vi "模拟量采集.vi"(11 "STOP 2":bool) -> (0 "压力2":dbl[](array[numeric]) format="%.2f", 1 "位移2":dbl[](array[numeric]) format="%.2f", 2 "压力1":dbl[](array[numeric]) format="%.2f", 3 "位移1":dbl[](array[numeric]) format="%.2f")   [LabVIEW 2010]
panel:
  out "CH0 15":dbl[](array[numeric]) format="%.2f"
  out "CH0 14":dbl[](array[numeric]) format="%.2f"
  out "CH0 13":dbl[](array[numeric]) format="%.2f"
  out "CH0 12":dbl[](array[numeric]) format="%.2f"
  out "CH0 11":dbl[](array[numeric]) format="%.2f"
  out "CH0 10":dbl[](array[numeric]) format="%.2f"
  out "CH0 9":dbl[](array[numeric]) format="%.2f"
  out "CH0 8":dbl[](array[numeric]) format="%.2f"
  out "CH0 7":dbl[](array[numeric]) format="%.2f"
  out "CH0 6":dbl[](array[numeric]) format="%.2f"
  out "CH0 5":dbl[](array[numeric]) format="%.2f"
  out "CH0 4":dbl[](array[numeric]) format="%.2f"
  # "±10V量程采集演示"
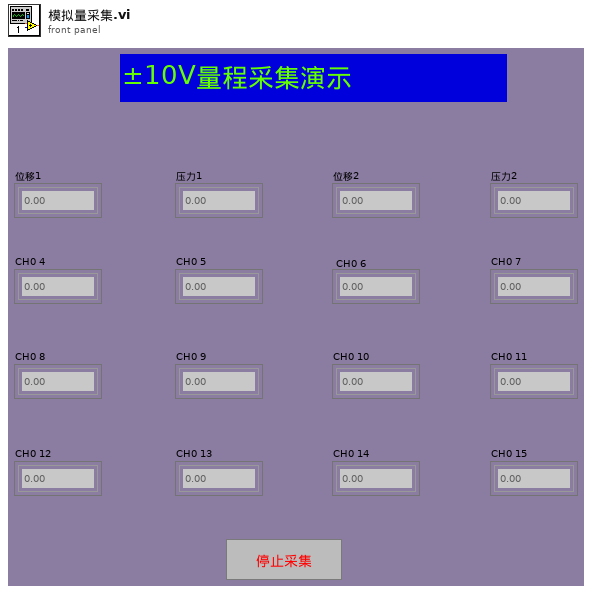
[diagram p1: front panel]
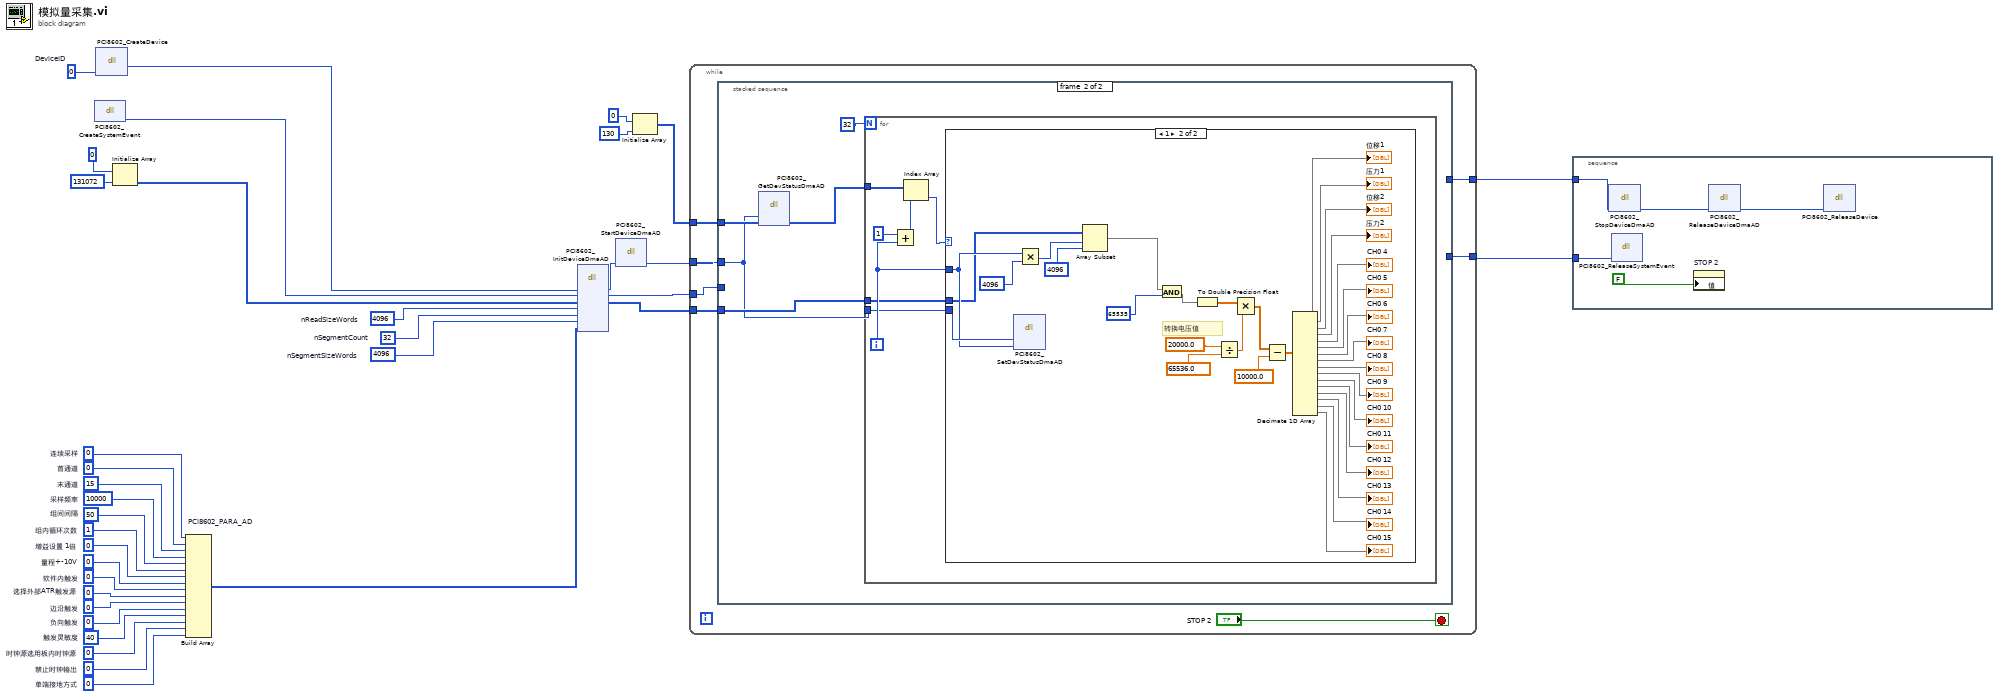
[diagram p0: block diagram]
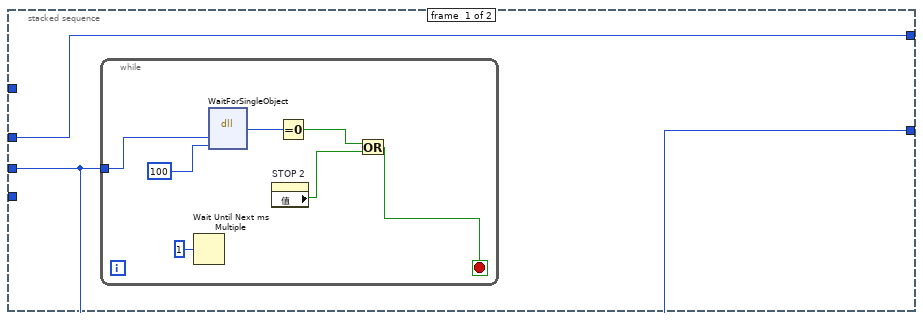
[diagram p2: hidden frame]
diagram:
  w1 = 0  # 单端接地方式
  w4 = 40  # 触发灵敏度
  w10 = 0  # 增益设置 1倍
  w11 = 1  # 组内循环次数
  w12 = 50  # 组间间隔
  w14 = 15  # 末通道
  w15 = 0  # 首通道
  w16 = 0  # 连续采样
  w2 = 0  # 禁止时钟输出
  w3 = 0  # 时钟源选用板内时钟源
  w5 = 0  # 负向触发
  w6 = 0  # 边沿触发
  w7 = 0  # 选择外部ATR触发源
  w8 = 0  # 软件内触发
  w9 = 0  # 量程+-10V
  w13 = 10000  # 采样频率
  w18 = 4096  # nSegmentSizeWords
  w19 = 32  # nSegmentCount
  w20 = 4096  # nReadSizeWords
  w28 = 0  # DeviceID
  n1 = dll-call lib="PCI8602" fn="PCI8602_CreateSystemEvent" label="CreateSystemEvent"() -> ("hEvent"=w22:i32)  [unwired: 3 in, 2 out]
  n2 = dll-call lib="PCI8602" fn="PCI8602_CreateDevice" label="CreateDevice"("DeviceID"=w28) -> (w23:i32)  [unwired: 4 in, 2 out]
  n3 = Initialize Array(u32 0, u32 131072 ("dimension size")) -> (w21:u32[])
  n4 = Build Array "PCI8602_PARA_AD"(w16, w15, w14, w13, w12, w11, w10, w9, w8, w7, w6, w5, w4, w3, w2, w1) -> (w17:i32[])
  n5 = dll-call lib="PCI8602" fn="PCI8602_InitDeviceDmaAD" label="InitDeviceDmaAD"("hDevice"=w23, "hDmaEvent"=w22, "ADBuffer"=w21, "nReadSizeWords"=w20, "nSegmentCount"=w19, "nSegmentSizeWords"=w18, "pADPara"=w17) -> ("hDevice"=w33:i32, "hDmaEvent"=w29:i32, "ADBuffer"=w31:u32[])  [unwired: 8 in, 2 out]
  n6 = dll-call lib="PCI8602" fn="PCI8602_StartDeviceDmaAD" label="StartDeviceDmaAD"("hDevice"=w33) -> ("hDevice"=w30:i32)  [unwired: 4 in, 2 out]
  n7 = Initialize Array(0 ("element"), 130 ("dimension size")) -> (w32:i32[])
  n8 = while {
    tunnel: w32 -> [w41]
    tunnel: w31 -> [w40]
    tunnel: w30 -> [w39]
    tunnel: [w38] -> w25
    tunnel: w29 -> [w37]
    tunnel: [w36] -> w24
    stop <- "STOP 2" stop-if-true
    n9 = stacked-sequence {
      tunnel: w41 -> [_ w53]
      tunnel: w40 -> [_ w55]
      tunnel: w39 -> [w44 w52]
      tunnel: [w44 _] -> w38
      tunnel: w37 -> [w43 _]
      tunnel: [w43 _] -> w36
      frame #0 {
        n10 = while {
          tunnel: w43 -> [w45]
          stop <- w46 stop-if-true
          n11 = Wait Until Next ms Multiple(millisecond multiple=u32 1) -> ()  [unwired: 1 out]
          n12 = dll-call lib="kernel32" fn="WaitForSingleObject"("hEvent"=w45, "dwMilliseconds"=100) -> (w49:u32)  [unwired: 5 in, 2 out]
          n13 = property on="STOP 2" class="Bool (严格)"() -> ("值"=w47:bool)  [unwired: 2 in, 2 out]
          n14 = Equal To 0?(x=w49) -> (x = 0?=w48:bool)
          n15 = Or(x=w48, y=w47) -> (x .or. y?=w46:bool)
        }
      }
      frame #1 {
        n16 = dll-call lib="PCI8602" fn="PCI8602_GetDevStatusDmaAD" label="GetDevStatusDmaAD"("hDevice"=w52, "pDMAStatus"=w53) -> ("pDMAStatus"=w54:i32[])  [unwired: 5 in, 2 out]
        n17 = for {
          N: 32 -> [_]
          tunnel: w54 -> [w63]
          tunnel: w52 -> [w58]
          tunnel: w55 -> [w57]
          i -> [w60]
          n18 = Add(x=1, y=w60) -> (x+y=w59:i32)
          n19 = Index Array(array=w63, index=w59) -> (element=w62:i32)
          n20 = case shown="1" w62 {
            tunnel: w60 -> [_ w91]
            tunnel: w58 -> [_ w92]
            tunnel: w57 -> [_ w65]
            frame 0, Default {
            }
            frame 1 {
              # "转换电压值"
              n21 = dll-call lib="PCI8602" fn="PCI8602_SetDevStatusDmaAD" label="SetDevStatusDmaAD"("hDevice"=w92, "iClrBufferID"=w91) -> ()  [unwired: 6 in, 2 out]
              n22 = Multiply(x=w91, y=4096) -> (x*y=w93:i32)
              n23 = Array Subset(array=w65, index=w93, length=4096) -> (w64:u32[])
              n24 = And(x=w64, y=65535) -> (x .and. y?=w82:u32[])
              n25 = To Double Precision Float(number=w82) -> (double precision float=w83:dbl[])
              n26 = Divide(x=20000.0, y=65536.0) -> (x/y=w86:dbl)
              n27 = Multiply(x=w83, y=w86) -> (x*y=w85:dbl[])
              n28 = Subtract(x=w85, y=10000.0) -> (x-y=w84:dbl[])
              n29 = Decimate 1D Array(w84) -> (→"位移1":dbl[], →"压力1":dbl[], →"位移2":dbl[], →"压力2":dbl[], →"CH0 4":dbl[], →"CH0 5":dbl[], →"CH0 6":dbl[], →"CH0 7":dbl[], →"CH0 8":dbl[], →"CH0 9":dbl[], →"CH0 10":dbl[], →"CH0 11":dbl[], →"CH0 12":dbl[], →"CH0 13":dbl[], →"CH0 14":dbl[], →"CH0 15":dbl[])
            }
          }
        }
      }
    }
  }
  n30 = stacked-sequence {
    tunnel: w25 -> [w98]
    tunnel: w24 -> [w97]
    frame #0 {
      n31 = dll-call lib="PCI8602" fn="PCI8602_StopDeviceDmaAD" label="StopDeviceDmaAD"("hDevice"=w98) -> ("hDevice"=w100:i32)  [unwired: 4 in, 2 out]
      n32 = dll-call lib="PCI8602" fn="PCI8602_ReleaseSystemEvent" label="ReleaseSystemEvent"("hEvent"=w97) -> ()  [unwired: 5 in, 2 out]
      n33 = property on="STOP 2" class="Bool (严格)"("值"=FALSE) -> ()  [unwired: 2 in, 2 out]
      n34 = dll-call lib="PCI8602" fn="PCI8602_ReleaseDeviceDmaAD" label="ReleaseDeviceDmaAD"("hDevice"=w100) -> ("hDevice"=w96:i32)  [unwired: 4 in, 2 out]
      n35 = dll-call lib="PCI8602" fn="PCI8602_ReleaseDevice" label="ReleaseDevice"("hDevice"=w96) -> ()  [unwired: 5 in, 2 out]
    }
  }
